vi "Clear.vi"(8 "error in (no error)":errorcluster, 11 "Text Log in":refnum<class "XML Log.lvclass">) -> (0 "error out":errorcluster, 2 "Error Log File Path":path, 3 "Text Log out":refnum<class "XML Log.lvclass">)   [LabVIEW 2020, in "Error Log Classes.lvlib" / "XML Log.lvclass"]
uses:
  XML Log.lvclass
  <resource>/objmgr/DOMUserDefRef.rc
  <vilib>/xml/NI_XML.lvlib
  <vilib>/xml/Close Reference(Node).vi
  <vilib>/xml/Close Reference(NdList).vi
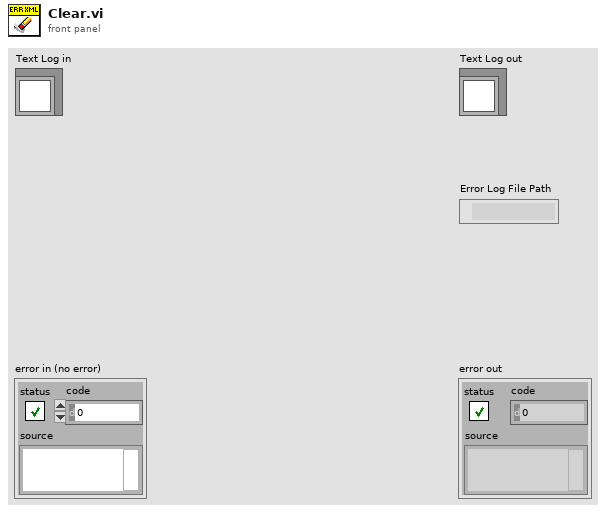
[diagram p1: front panel]
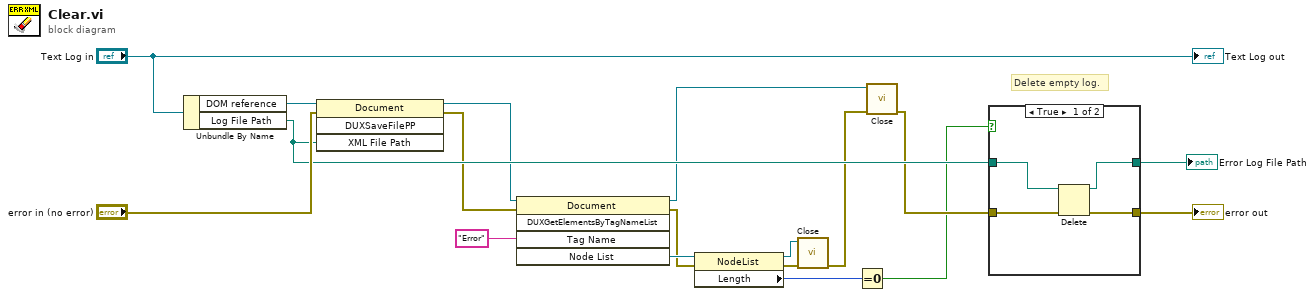
[diagram p0: block diagram]
diagram:
  # "Delete empty log."
  n1 = Unbundle By Name("Text Log in") -> ("DOM reference"=w17:refnum<k20>, "Log File Path"=w14:path)
  n2 = invoke class="Document" method="DUXSaveFilePP"(reference=w17, error in="error in (no error)", "XML File Path"=w14) -> (reference out=w9:refnum<k20>, error out=w8:errorcluster)  [unwired: 1 in, 2 out]
  n3 = invoke class="Document" method="DUXGetElementsByTagNameList"(reference=w9, error in=w8, "Tag Name"="Error") -> (reference out=w2:refnum<k20>, error out=w10:errorcluster, "Node List"=w11:refnum<k20>)  [unwired: 2 in, 2 out]
  n4 = property class="NodeList"(reference=w11, error in=w10) -> (reference out=w3:refnum<k20>, error out=w4:errorcluster, "Length"=w6:i32)
  n5 = call-poly <vilib>:"Close.vi"("error in (no error)"=w4, "node list"=w3) -> ("error out"=w1:errorcluster)  [unwired: 7 in]
  n6 = Equal To 0?(x=w6) -> (x = 0?=w5:bool)
  n7 = call-poly <vilib>:"Close.vi"("error in (no error)"=w1, "node"=w2) -> ("error out"=w13:errorcluster)  [unwired: 7 in]
  n8 = case shown="True" w5 {
    tunnel: w13 -> [w22 w24]
    tunnel: [w21 w24] -> w15
    tunnel: w14 -> [w20 w23]
    tunnel: [w19 w23] -> w12
    frame True {
      n9 = Delete(path (use dialog)=w20, error in=w22) -> (deleted path=w19:path, error out=w21:errorcluster)  [unwired: 3 in, 1 out]
    }
    frame False {
    }
  }
  "error out" <- w15
  "Error Log File Path" <- w12
  "Text Log out" <- "Text Log in"
